vi "Holding Register Get Mapping.vi"(8 "error in (no error)":errorcluster, 11 "Item Ref in":T1 format="%.0x") -> (0 "error out":errorcluster, 2 "Mapping":T2 {"VS Reference" format="%.0x"}, 3 "Item Ref out":T1 format="%.0x")   [LabVIEW 2021]
uses:
  Shared/Controls/Data Model/DataType.ctl
  Shared/Modbus Master Shared.lvlib
  Shared/Controls/Data Model/Mapping.ctl
  <vilib>/NI VeriStand/Custom Device API/Custom Device Item Ref.ctl
  <vilib>/NI VeriStand/Custom Device API/Custom Device API.lvlib
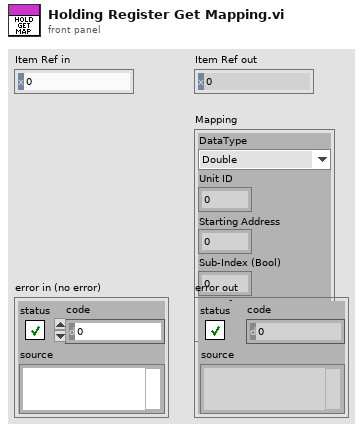
[diagram p1: front panel]
types:
  T1 = typedef "Custom Device API.lvlib/Custom Device Item Ref.ctl" = u64
  T2 = typedef "Modbus Master Shared.lvlib/Mapping.ctl" = cluster{"DataType":T3, "Unit ID":u8, "Starting Address":u16, "Sub-Index (Bool)":u16, "VS Reference":T1}
  T3 = typedef "Modbus Master Shared.lvlib/DataType.ctl" = enum16{"Double", "Single", "I64", "I32", "I16", "I8", "U64", "U32", "U16", "U8", "Boolean"}
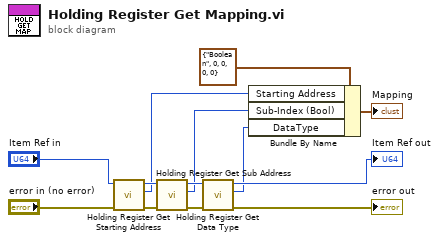
[diagram p0: block diagram]
diagram:
  n1 = call "Holding Register Get Starting Address.vi"("error in (no error)"="error in (no error)", "Item Ref in"="Item Ref in") -> ("error out"=w10:errorcluster, "Value"=w3:u16, "Item Ref out"=w11:T1)  [unwired: 7 in]
  n2 = call "Holding Register Get Sub Address.vi"("error in (no error)"=w10, "Item Ref in"=w11) -> ("error out"=w8:errorcluster, "Value"=w2:u16, "Item Ref out"=w9:T1)  [unwired: 7 in]
  n3 = call "Holding Register Get Data Type.vi"("error in (no error)"=w8, "Item Ref in"=w9) -> ("error out"=→"error out":errorcluster, "Data Type"=w1:T3, "Item Ref out"=→"Item Ref out":T1)  [unwired: 7 in]
  n4 = Bundle By Name(cluster=T2 {"DataType"=enum."Boolean", "Unit ID"=0, "Starting Address"=0, "Sub-Index (Bool)"=0, "VS Reference"=0} ("Mapping"), "Starting Address"=w3, "Sub-Index (Bool)"=w2, "DataType"=w1) -> (→"Mapping":T2)
